vi "ScriptCreateIOselector.vi"(4 "numeric representation":T1=enum."Word", 6 "digital(F)/numeric(T)":bool, 7 "indicator (F)/control (T)":bool, 8 "error in (no error)":errorcluster, 9 "IO names":string[](array[string]), 10 "VI path":path, 11 "Application in":refnum<vi>) -> ()   [LabVIEW 2014]
uses:
  <vilib>/numeric/LVNumericRepresentation.ctl
  <vilib>/eio/EIO_TerminalDirection.ctl
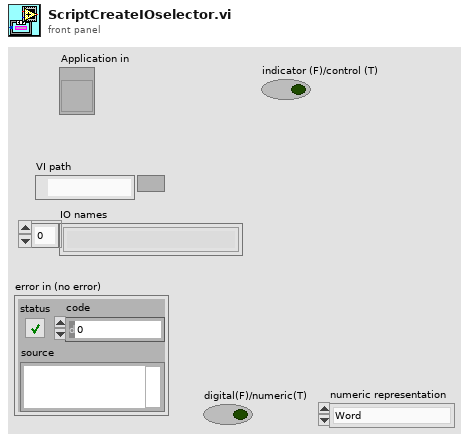
[diagram p1: front panel]
types:
  T1 = typedef "LVNumericRepresentation.ctl" = enum32{"Extended Precision", "Double Precision", "Single Precision", "Long", "Word", "Byte", "Unsigned Long", "Unsigned Word", "Unsigned Byte", "Complex Extended", "Complex Double", "Complex Single", "Quad", "Unsigned Quad", "Fixed-Point"}
  T2 = typedef "EIO_TerminalDirection.ctl" = enum16{"read", "write", "none", "both"}
  T3 = typedef "LVPositionTypeDef.ctl" = cluster{"Left":i32, "Top":i32}
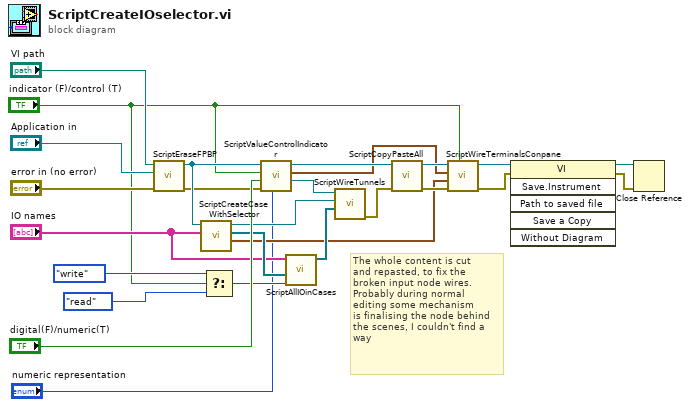
[diagram p0: block diagram]
diagram:
  # "The whole content is cut\nand repasted, to fix the\nbroken input node wires.\nProbably during normal\nediting some mechanism\nis finalising the node behind\nthe scenes, I couldn't find a\nway"
  n1 = call "ScriptEraseFPBP.vi"("error in (no error)"="error in (no error)", "application reference (local)"="Application in", "VI path"="VI path") -> ("error out"=w15:errorcluster, "VI out"=w22:refnum<vi>)  [unwired: 7 in]
  n2 = call "ScriptCreateCaseWithSelector.vi"("I/O names"="IO names", "VI in"=w22) -> ("Enum position"=w3:T3, "Case diagrams"=w19:refnum<vi>[], "CaseStructure out"=w20:refnum<vi>)  [unwired: 6 in, 1 out]
  n3 = Select(t=EIO_TerminalDirection."write" ("direction"), s="indicator (F)/control (T)", f=EIO_TerminalDirection."read" ("direction")) -> (s? t:f=w12:T2)
  n4 = call "ScriptValueControlIndicator.vi"("numeric representation"="numeric representation", "error in (no error)"=w15, "digital(F)/numeric(T)"="digital(F)/numeric(T)", "indicator (F)/control (T)"="indicator (F)/control (T)", "VI in"=w22) -> ("Value terminal"=w9:refnum<vi>, "Value position"=w2:T3, "VI out"=w11:refnum<vi>)  [unwired: 3 in, 1 out]
  n5 = call "ScriptAllIOinCases.vi"("direction"=w12, "Case diagrams"=w19, "I/O names"="IO names") -> ("IO terminals"=w21:refnum<vi>[])  [unwired: 8 in]
  n6 = call "ScriptWireTunnels.vi"("i/o terminals"=w21, "CaseStructure in"=w20, "ControlTerminal in"=w9) -> ("error out"=w10:errorcluster)  [unwired: 8 in]
  n7 = call "ScriptCopyPasteAll.vi"("error in (no error)"=w10, "VI in"=w11) -> ("error out"=w7:errorcluster, "VI out"=w6:refnum<vi>)  [unwired: 8 in]
  n8 = call "ScriptWireTerminalsConpane.vi"("indicator (F)/control (T)"="indicator (F)/control (T)", "error in (no error)"=w7, "Enum position"=w3, "Value position"=w2, "VI in"=w6) -> ("error out"=w4:errorcluster, "VI out"=w5:refnum<vi>)  [unwired: 5 in]
  n9 = invoke class="VI" method="Save.Instrument"(reference=w5, error in=w4) -> (reference out=w16:refnum<vi>, error out=w17:errorcluster)  [unwired: 4 in, 4 out]
  n10 = Close Reference(reference=w16, error in (no error)=w17) -> ()  [unwired: 1 out]
